vi "rad_Target Info Dialog.vi"(11 "Target Information":T1={"Hostname"="", "Serial number"="", "Product name"="", "Product code"=0, "System status"="", "Credential type"=enum."None/Unlocked", "User added?"=FALSE, "Primary NIC"={"MAC address"="", "IP Address Request Mode"=2, "IP address"="", "Subnet mask"="", "Gateway"="", "DNS server"=""}} {"Primary NIC"."IP Address Request Mode" items=["Static"=1, "DHCP/Link-Local"=2, "Link-Local Only"=4, "DHCP Only"=8]}) -> ()   [LabVIEW 2020]
uses:
  support/New folder/Target Information.ctl
  TypeDefs/rad_Target Network Settings.ctl
panel:
  in  "ViewInstalledSoftware":bool
  out "Target Information":string[][](table)
  in  "Close":bool
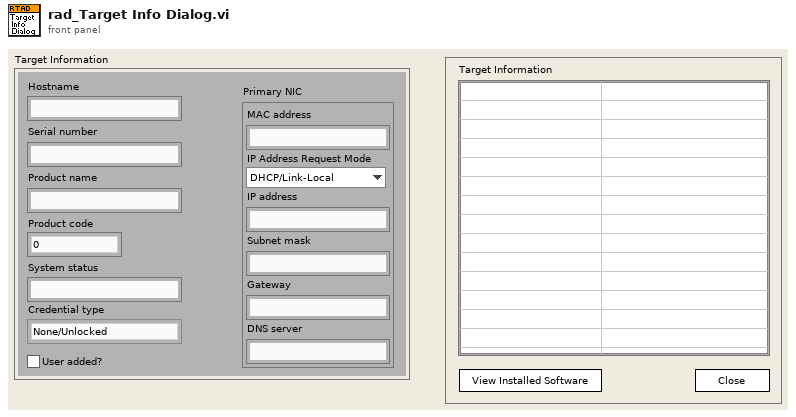
[diagram p1: front panel]
types:
  T1 = typedef "Target Information.ctl" = cluster{"Hostname":string, "Serial number":string, "Product name":string, "Product code":i32, "System status":string, "Credential type":enum16{"None/Unlocked", "FTP Password", "NIAuth Credentials"}, "User added?":bool, "Primary NIC":T2}
  T2 = typedef "rad_Target Network Settings.ctl" = cluster{"MAC address":string, "IP Address Request Mode":i32, "IP address":string, "Subnet mask":string, "Gateway":string, "DNS server":string}
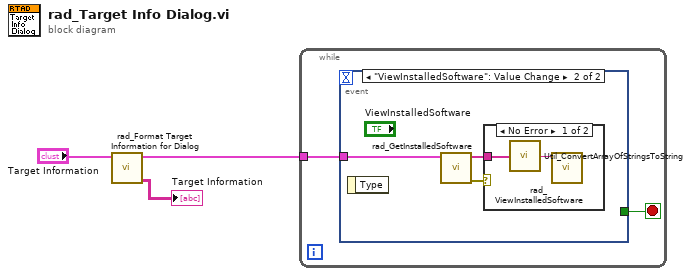
[diagram p0: block diagram]
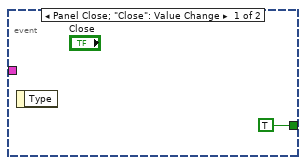
[diagram p2: hidden frame]
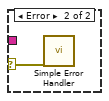
[diagram p3: hidden frame]
diagram:
  n1 = call "rad_Format Target Information for Dialog.vi"("target settings in"="Target Information") -> ("Target Information"=→"Target Information":string[][], "target settings out"=w1:T1)  [unwired: 9 in]
  n2 = while {
    tunnel: w1 -> [w4]
    stop <- w5 stop-if-true
    n3 = event shown="[1] \"ViewInstalledSoftware\": Value Change" {
      selector: _ -> [_ _]
      dyn-events: _ -> [_ _]
      timeout: _ -> [_ _]
      tunnel: [TRUE _] -> w5
      tunnel: w4 -> [_ w8]
      event Panel Close; "Close": Value Change {
        n4 = event-data() -> ()  [unwired: 1 in, 1 out]
      }
      event "ViewInstalledSoftware": Value Change {
        n5 = event-data() -> ()  [unwired: 1 in, 1 out]
        n6 = call "rad_GetInstalledSoftware.vi"("Target settings"=w8) -> ("error out"=w7:errorcluster, "installedSoftware"=w9:string[])  [unwired: 9 in]
        n7 = case shown="No Error" w7 {
          selector: w7 -> [_ w12]
          tunnel: w9 -> [w10 _]
          frame No Error {
            n8 = call "Util_ConvertArrayOfStringsToString.vi"("Array<string>"=w10) -> ("String"=w11:string)
            n9 = call "rad_ViewInstalledSoftware.vi"("Installed Software"=w11) -> ()  [unwired: 11 in]
          }
          frame Error {
            n10 = call <vilib>:"Simple Error Handler.vi"("error in (no error)"=w12) -> ()  [unwired: 4 in, 5 out]
          }
        }
      }
    }
  }
